vi "onCreated.vi"(8 "error in (no error)":errorcluster, 11 "SMU":refnum<class "SMU.lvclass">) -> (0 "error out":errorcluster, 3 "SMU out":refnum<class "SMU.lvclass">)   [LabVIEW 2017, in "SMU.lvclass"]
doc: "JKI State Machine Objects (SMO) 1.3.0.56\nJKI - JKI\nCopyright (c) 2017, JKI"
uses:
  SMU.lvclass
  D:/Program Files (x86)/National Instruments/LabVIEW 2017/vi.lib/JKI/JKI SMO/SMO/SMO.lvclass
  D:/upwork/Laser Measurement Tool/Laser/project/Subsystems/MeasuringDevice/MeasuringDevice.lvclass
  CircularBuffer/types/type.DBL/type.DBL.lvclass
  D:/upwork/Laser Measurement Tool/Laser/project/Subsystems/CircularBuffer/types/type/type.lvclass
  MeasuringDevice/MeasuringDevice.lvclass
  CircularBuffer/CircularBuffer.lvclass
  <vilib>/JKI/JKI SMO/SMO/SMO.lvclass
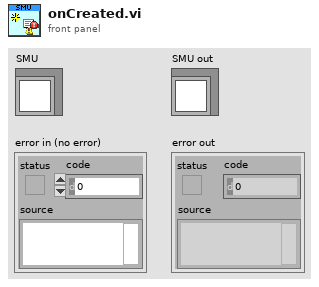
[diagram p1: front panel]
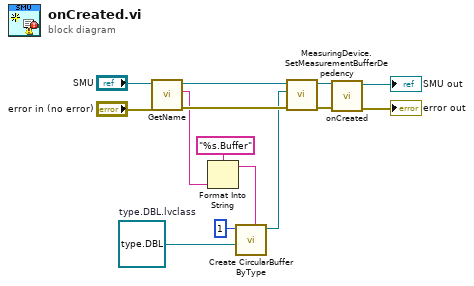
[diagram p0: block diagram]
diagram:
  w9 = refnum<class "type.DBL.lvclass"> refnum  # type.DBL.lvclass
  n1 = call <vilib>:"GetName.vi"("error in (no error)"="error in (no error)", "SMO"="SMU") -> ("error out"=w7:errorcluster, "Name"=w3:string, "SMO out"=w8:refnum<class "SMU.lvclass">)  [unwired: 7 in]
  n2 = Format Into String(format string="%s.Buffer", w3) -> (resulting string=w4:string)  [unwired: 2 in, 1 out]
  n3 = call "Create CircularBuffer ByType.vi"("Buffer Name"=w4, "type"=w9, "BufferSize"=1) -> ("CircularBuffer out"=w6:refnum<class "CircularBuffer.lvclass">)  [unwired: 6 in, 2 out]
  n4 = call "MeasuringDevice.SetMeasurementBufferDepedency.vi"("error in (no error)"=w7, "CircularBuffer"=w6, "MeasuringDevice"=w8) -> ("error out"=w11:errorcluster, "MeasuringDevice"=w12:refnum<class "SMU.lvclass">)  [unwired: 7 in]
  n5 = call-parent "onCreated.vi"("error in (no error)"=w11, "SMO"=w12) -> ("error out"=→"error out":errorcluster, "SMO out"=→"SMU out":refnum<class "SMU.lvclass">)  [unwired: 8 in]
